vi "ESC Per Block Plugin.vi"() -> (5 "Plug in titles":string[](array[string]), 7 "Plug in values":string[](array[string]))   [LabVIEW 2022 SP3]
uses:
  Controls/Post_Process.ctl
  <vilib>/Analysis/baseanly.llb/Mean (DBL).vi
  Globals/Meas_global.vi
  <vilib>/measure/matone.llb/Extract Single Tone Information 1 Chan.vi
  <vilib>/measure/NI_MAPro.lvlib
  <vilib>/Analysis/NI_AALBase.lvlib
panel:
  in  "Blades/Poles":i32[](array[numeric])
  in  "Freq Channels":i32[](array[numeric])
  out "detected frequency":dbl format="%.2p"
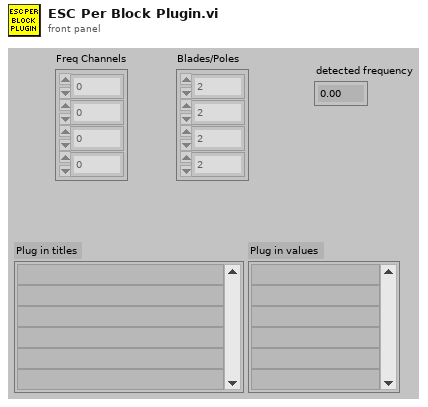
[diagram p1: front panel]
types:
  T1 = typedef "Setup.ctl" = enum16{"Run Program", "Show Setup", "Save Current Setup", "Setup Front Panel"}
  T2 = typedef "Post_Process.ctl" = enum16{"Take New Data", "Post Process Raw Data File"}
  T3 = typedef "Analysis_info_cluster.ctl" = cluster{"Colour":u32, "Inst type":T4, "Inst name":string, "Symbol":string, "Code name":string, "Extra Info":string, "Inst Array":T5, "Extra Titles":string[], "Extra Values":string[], "U":dbl, "u^2":dbl, "u^3":dbl, "u^4":dbl, "Skew_u":dbl, "Kurt_u":dbl, "Sd Error in Mean":dbl, "% u'/U":dbl, "X":dbl, "Y":dbl, "Z":dbl, "Timescale integral Estimate":dbl, "Sd Error in Variance":dbl, "Calib File":path, "Calib Constants":dbl[], "Output Position":bool, "Stats":enum16{"None", "Basic", "Full"}, "Av Sampling Rate":dbl, "Av No of Samples":dbl, "Total Meas Time (s)":dbl, "ADAM Ch Name":string, "Max value":dbl, "Min value":dbl, "Req Sample Rate Hz":dbl, "Sync Delay Time (s)":dbl, "Ch No":i16, "Device":string, "Use Latest Calib":bool, "Port":string, "Metadata Ch Names":string[], "Metadata Ch Values":string[], "Label":string}
  T4 = typedef "Inst_type.ctl" = enum16{"Raw voltage", "Raw with zero offsetting", "Propeller anemometer", "Pressure Transducer", "Pitot-static tube", "Hot wire", "Cross wire 1", "Cross wire 2", "Generic Linear", "Generic Polynomial", "Generic BackPoly", "Fast FID", "Thermocouple", "Cold wire", "Pulsed Wire", "LDA Vel", "LDA Tran time", "LDA Arr time", "Microphone"}
  T5 = typedef "Instrument_Array.ctl" = enum16{"PWA", "LDA", "Analogue"}
  T6 = typedef "Time_Trace_Cluster.ctl" = cluster{"Weighting":dbl[], "Voltage":dbl[], "Eng Values":dbl[]}
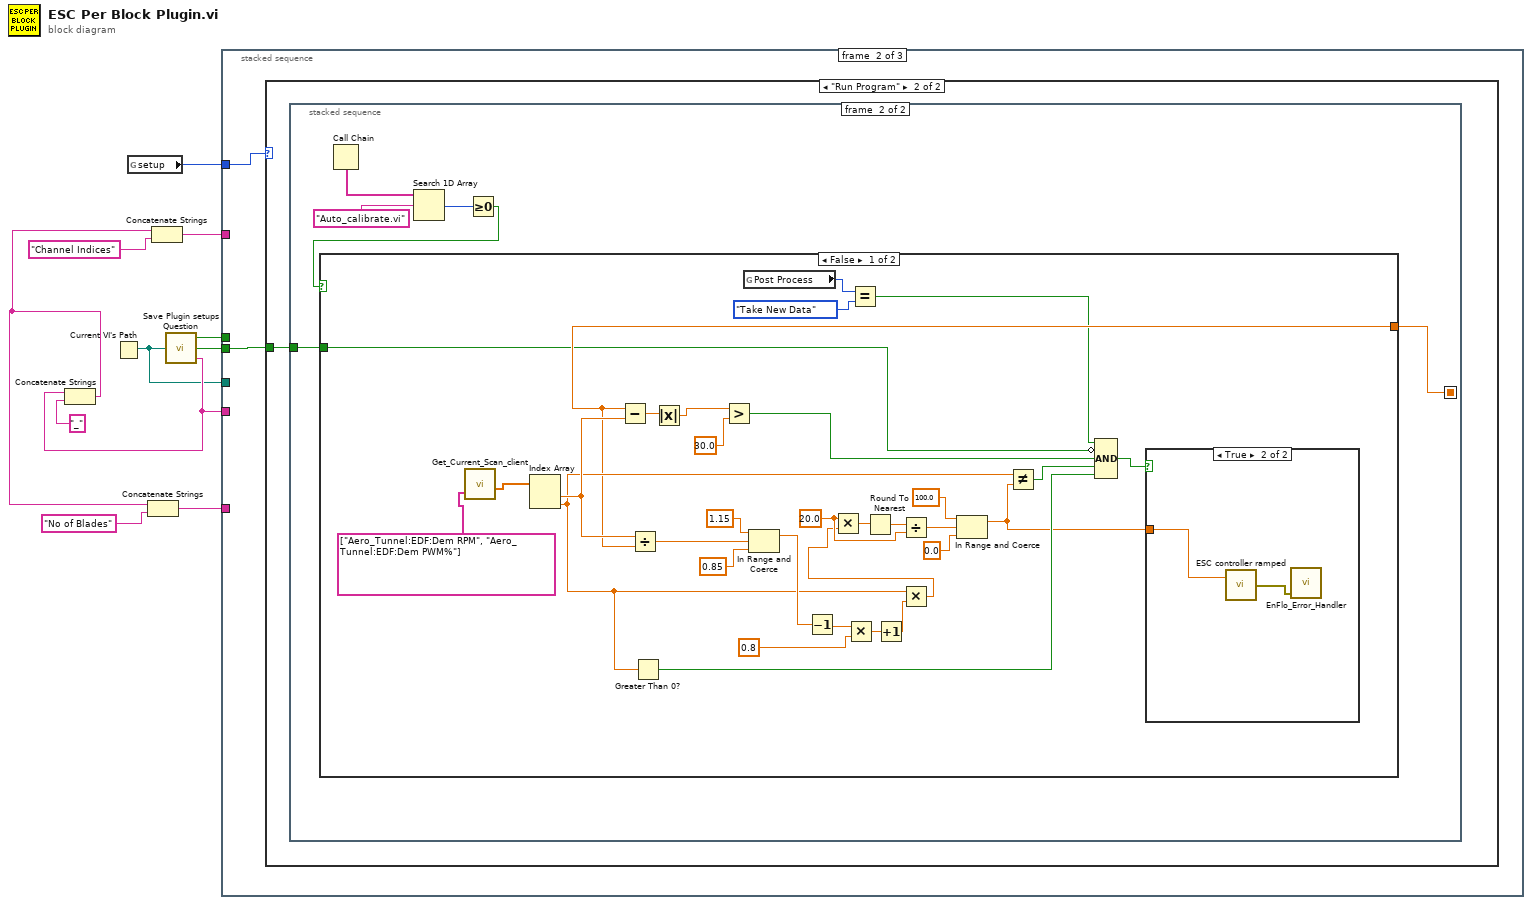
[diagram p0: block diagram]
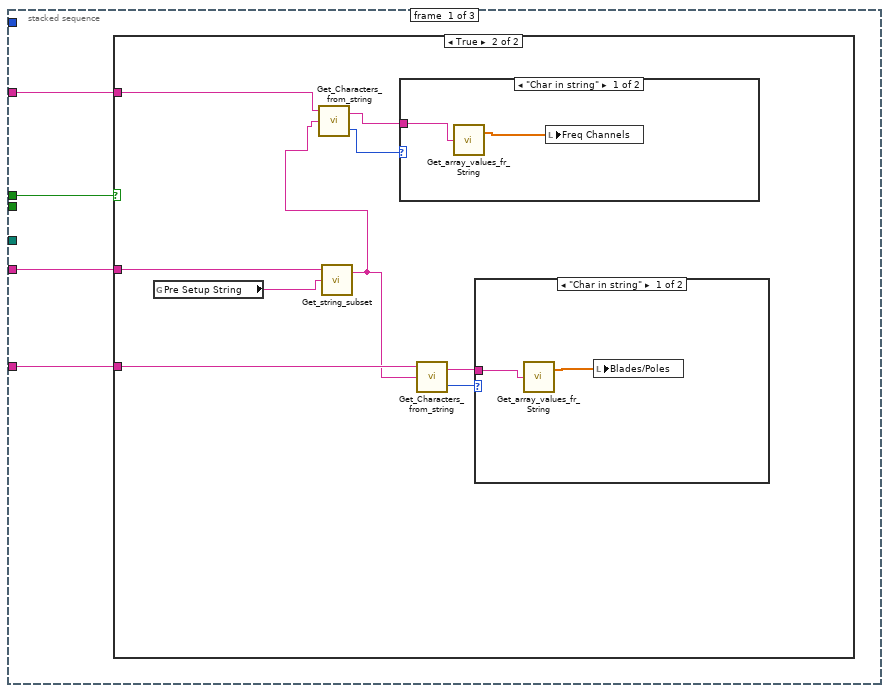
[diagram p2: hidden frame]
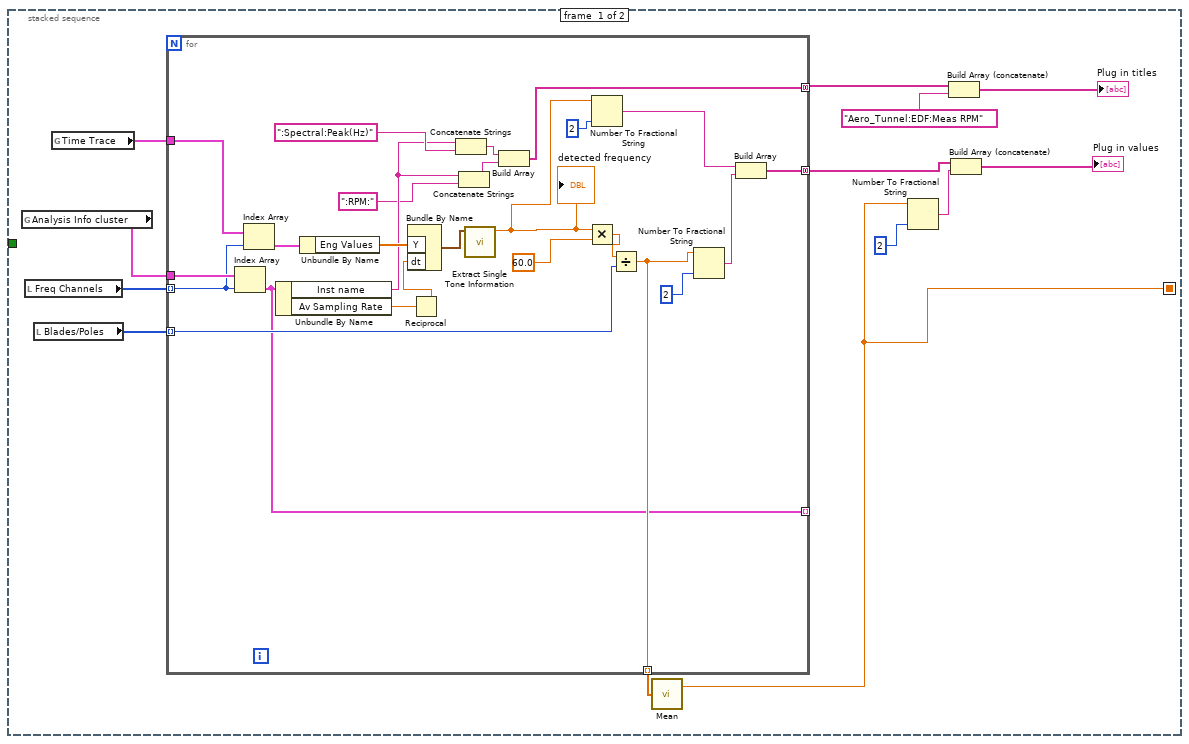
[diagram p7: hidden frame]
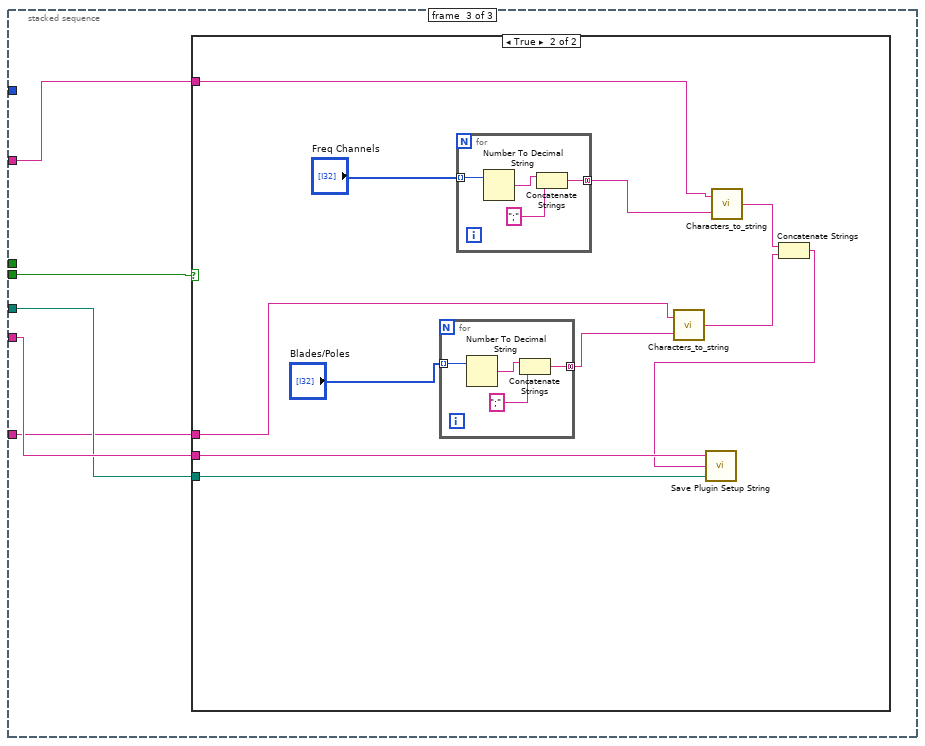
[diagram p10: hidden frame]
diagram:
  n1 = Current VI's Path() -> (path=w5:path)
  n2 = global read "Meas_global.vi" "setup"() -> (w1:T1)
  n3 = call "Save Plugin setups Question.vi"("VI path"=w5) -> ("Load Plugin Setup"=w11:bool, "Save Plugin Setup"=w6:bool, "Plugin_Label"=w7:string)
  n4 = Concatenate Strings(w7, "_" ("string")) -> (w3:string)
  n5 = Concatenate Strings(w3, "No of Blades" ("Label for value")) -> (w2:string)
  n6 = Concatenate Strings(w3, "Channel Indices" ("Label for value")) -> (w8:string)
  n7 = stacked-sequence {
    tunnel: w11 -> [w15 _ _]
    tunnel: w8 -> [w14 _ w112]
    tunnel: w7 -> [w13 _ w113]
    tunnel: w6 -> [_ w29 w114]
    tunnel: w5 -> [_ _ w111]
    tunnel: w2 -> [w12 _ w110]
    tunnel: w1 -> [_ w30 _]
    frame #0 {
      n8 = case shown="True" w15 {
        tunnel: w14 -> [_ w19]
        tunnel: w13 -> [_ w23]
        tunnel: w12 -> [_ w22]
        frame False {
        }
        frame True {
          n9 = global read "Meas_global.vi" "Pre Setup String"() -> (w24:string)
          n10 = call "Get_string_subset.vi"("String to split"=w24, "File Label"=w23) -> ("Output string"=w18:string)  [unwired: 2 in, 1 out]
          n11 = call "Get_Characters_from_string.vi"("Input string"=w18, "Variable name"=w19) -> ("Status"=w16:enum16{"Char in string", "Char not in string"}, "Value"=w17:string)  [unwired: 1 in]
          n12 = case shown="\"Char in string\"" w16 {
            tunnel: w17 -> [w28 _]
            frame "Char in string" {
              n13 = call "Get_array_values_fr_String.vi"("String Value"=w28) -> ("Numeric Array"=w27:dbl[])  [unwired: 1 out]
              n14 = local write "Freq Channels"(w27) -> ()
            }
            frame "Char not in string" {
            }
          }
          n15 = call "Get_Characters_from_string.vi"("Input string"=w18, "Variable name"=w22) -> ("Status"=w21:enum16{"Char in string", "Char not in string"}, "Value"=w20:string)  [unwired: 1 in]
          n16 = case shown="\"Char in string\"" w21 {
            tunnel: w20 -> [w26 _]
            frame "Char in string" {
              n17 = call "Get_array_values_fr_String.vi"("String Value"=w26) -> ("Numeric Array"=w25:dbl[])  [unwired: 1 out]
              n18 = local write "Blades/Poles"(w25) -> ()
            }
            frame "Char not in string" {
            }
          }
        }
      }
    }
    frame #1 {
      n19 = case shown="\"Run Program\"" w30 {
        tunnel: w29 -> [_ w31]
        frame Default {
        }
        frame "Run Program" {
          n20 = stacked-sequence {
            seq-local: [w37 _] -> [_ w75]
            tunnel: w31 -> [_ w74]
            frame #0 {
              n21 = global read "Meas_global.vi" "Analysis Info cluster"() -> (w35:T3[])
              n22 = local read "Freq Channels"() -> (w44:i32[])
              n23 = local read "Blades/Poles"() -> (w43:i32[])
              n24 = global read "Meas_global.vi" "Time Trace"() -> (w36:T6[])
              n25 = for {
                tunnel: [w69] -> w41 mode=concatenating
                tunnel: [w68] -> w42 mode=indexing
                tunnel: w36 -> [w67]
                tunnel: w35 -> [w66]
                tunnel: w44 -> [w65] mode=indexing
                tunnel: w43 -> [w64] mode=indexing
                tunnel: [w63] -> w39 mode=concatenating
                tunnel: [w62] -> _ mode=indexing
                n26 = Index Array(array=w66, index=w65) -> (element=w62:T3)
                n27 = Index Array(array=w67, index=w65) -> (element=w55:T6)
                n28 = Unbundle By Name(w62) -> ("Inst name"=w48:string, "Av Sampling Rate"=w53:dbl)
                n29 = Unbundle By Name(w55) -> ("Eng Values"=w54:dbl[])
                n30 = Reciprocal(x=w53) -> (1/x=w52:dbl)
                n31 = Bundle By Name("Y"=w54, "dt"=w52) -> (w51:waveform(dbl))  [unwired: 1 in]
                n32 = Concatenate Strings(w48, ":Spectral:Peak(Hz)" ("string")) -> (w46:string)
                n33 = Concatenate Strings(w48, ":RPM:" ("string")) -> (w45:string)
                n34 = call-poly <vilib>:"Extract Single Tone Information.vi"("time signal in"=w51) -> ("detected frequency"=w50:dbl)  [unwired: 5 in, 5 out]
                "detected frequency" <- w50
                n35 = Build Array(w46, w45) -> (w63:string[])
                n36 = Multiply(x=w50, y=60.0) -> (x*y=w59:dbl)
                n37 = Number To Fractional String(number=w50, precision (6)=i16 2) -> (F-format string=w58:string)  [unwired: 2 in]
                n38 = Divide(x=w59, y=w64) -> (x/y=w68:dbl)
                n39 = Number To Fractional String(number=w68, precision (6)=i16 2) -> (F-format string=w56:string)  [unwired: 2 in]
                n40 = Build Array(w58, w56) -> (w69:string[])
              }
              n41 = call-poly <vilib>:"Mean.vi"("X"=w42) -> ("mean"=w37:dbl)  [unwired: 1 out]
              n42 = Number To Fractional String(number=w37, precision (6)=i16 2) -> (F-format string=w33:string)  [unwired: 2 in]
              n43 = Build Array (concatenate)(w39, "Aero_Tunnel:EDF:Meas RPM" ("string")) -> (→"Plug in titles":string[])
              n44 = Build Array (concatenate)(w41, w33) -> (→"Plug in values":string[])
            }
            frame #1 {
              n45 = Call Chain() -> (call chain=w73:string[])
              n46 = Search 1D Array(1D array=w73, element="Auto_calibrate.vi") -> (index of element=w71:i32)  [unwired: 1 in]
              n47 = Greater Or Equal To 0?(x=w71) -> (x >= 0?=w70:bool)
              n48 = case shown="False" w70 {
                tunnel: w75 -> [w81 _]
                tunnel: w74 -> [w80 _]
                frame False {
                  w90 = 20.0 ("x")
                  n49 = call "Get_Current_Scan_client.vi"("multipleChannels"=string[] ["Aero_Tunnel:EDF:Dem RPM", "Aero_Tunnel:EDF:Dem PWM%"]) -> ("Numerical Values"=w100:dbl[])  [unwired: 1 in, 3 out]
                  n50 = Index Array(array=w100) -> (element #1=w97:dbl, element #2=w87:dbl)  [unwired: 2 in]
                  n51 = Subtract(x=w81, y=w97) -> (x-y=w96:dbl)
                  n52 = Divide(x=w97, y=w81) -> (x/y=w99:dbl)
                  n53 = Greater Than 0?(x=w87) -> (x > 0?=w86:bool)
                  n54 = Absolute Value(x=w96) -> (abs(x)=w95:dbl)
                  n55 = Greater?(x=w95, y=30.0) -> (0:w94:bool)
                  n56 = global read "Meas_global.vi" "Post Process"() -> (w78:T2)
                  n57 = In Range and Coerce(upper limit=1.15, x=w99, lower limit=0.85) -> (coerced(x)=w104:dbl)  [unwired: 1 out]
                  n58 = Decrement(x=w104) -> (x-1=w105:dbl)
                  n59 = Multiply(x=w105, y=0.8 ("upper limit")) -> (x*y=w106:dbl)
                  n60 = Equal?(x=w78, y=Post_Process."Take New Data" ("Post Process")) -> (x = y?=w77:bool)
                  n61 = Increment(x=w106) -> (x+1=w107:dbl)
                  n62 = Multiply(x=w87, y=w107) -> (x*y=w88:dbl)
                  n63 = Multiply(x=w90, y=w88) -> (x*y=w92:dbl)
                  n64 = Round To Nearest(number=w92) -> (nearest integer value=w91:dbl)
                  n65 = Divide(x=w91, y=w90) -> (x/y=w85:dbl)
                  n66 = In Range and Coerce(upper limit=100.0, x=w85, lower limit=0.0) -> (coerced(x)=w82:dbl)  [unwired: 1 out]
                  n67 = Not Equal?(x=w87, y=w82) -> (x != y?=w89:bool)
                  n68 = Compound Arithmetic op=AND(w77, invert w80, w94, w89, w86) -> (w93:bool)
                  n69 = case shown="True" w93 {
                    tunnel: w82 -> [_ w109]
                    frame False {
                    }
                    frame True {
                      n70 = call "ESC controller ramped.vi"("Output %"=w109) -> ("Error out"=w108:errorcluster)  [unwired: 2 in]
                      n71 = call "EnFlo_Error_Handler.vi"("error in (no error)"=w108) -> ()  [unwired: 3 in, 2 out]
                    }
                  }
                }
                frame True {
                }
              }
            }
          }
        }
      }
    }
    frame #2 {
      n72 = case shown="True" w114 {
        tunnel: w113 -> [_ w125]
        tunnel: w112 -> [_ w122]
        tunnel: w111 -> [_ w124]
        tunnel: w110 -> [_ w118]
        frame False {
        }
        frame True {
          n73 = for {
            tunnel: "Blades/Poles" -> [w129] mode=indexing
            tunnel: [w126] -> w117 mode=concatenating
            n74 = Number To Decimal String(number=w129) -> (decimal integer string=w128:string)  [unwired: 1 in]
            n75 = Concatenate Strings(w128, ";") -> (w126:string)
          }
          n76 = for {
            tunnel: "Freq Channels" -> [w133] mode=indexing
            tunnel: [w130] -> w121 mode=concatenating
            n77 = Number To Decimal String(number=w133) -> (decimal integer string=w132:string)  [unwired: 1 in]
            n78 = Concatenate Strings(w132, ";") -> (w130:string)
          }
          n79 = call "Characters_to_string.vi"("Characters to write"=w117, "Label for characters"=w118) -> ("Output string"=w116:string)  [unwired: 1 in]
          n80 = call "Characters_to_string.vi"("Characters to write"=w121, "Label for characters"=w122) -> ("Output string"=w120:string)  [unwired: 1 in]
          n81 = Concatenate Strings(w120, w116) -> (w123:string)
          n82 = call "Save Plugin Setup String.vi"("Plug In Pathname"=w124, "Setup String to Save"=w123, "PlugIn Label"=w125) -> ()  [unwired: 1 in, 1 out]
        }
      }
    }
  }
